vi "Initialize Control.vi"(8 "error in (no error)":errorcluster, 11 "DataGrid in":refnum<class "DataGrid.lvclass">) -> (0 "error out":errorcluster, 3 "DataGrid out":refnum<class "DataGrid.lvclass">)   [LabVIEW 2018, in "DataGrid.lvclass"]
doc: "The <b>Initialize VI</b> is a dynamic dispatch VI that must be overwritten in every QControl Class. It must <b>Call Parent Method</b> so that it recursively calls the initialize routine all of the way up the inheritance hierarchy. \n\nThe top most call is to the <b>Initialize Control VI</b> in Control.lvclass. This is the VI that starts the <b>Event Handler VI</b> if there was one overwritten in the QControl.\n<b> </b> <b> </b>\n©2016 Q Software Innovations, LLC (QSI)\nwritten by Quentin Alldredge\nproduced in LabVIEW 2015\n\nsupport@qsoftwareinnovations.com\nwww.qsoftwareinnovations.com\n\nAll rights reserved.\n\nRedistribution and use in source and binary forms, with or without modification, are permitted provided that the following conditions are met:\n\n * Redistributions of source code must retain the above copyright notice, this list of conditions and the following disclaimer.\n * Redistributions in binary form must reproduce the above copyright notice, this list of conditions and the following disclaimer in the documentation and/or other materials provided with the distribution.\n * Neither the name of Q Software Innovations, LLC. nor the names of its contributors may be used to endorse or promote products derived from this software without specific prior written permission.\n\nTHIS SOFTWARE IS PROVIDED BY THE COPYRIGHT HOLDERS AND CONTRIBUTORS \"AS IS\" AND ANY EXPRESS OR IMPLIED WARRANTIES, INCLUDING, BUT NOT LIMITED TO, THE IMPLIED WARRANTIES OF MERCHANTABILITY AND FITNESS FOR A PARTICULAR PURPOSE ARE DISCLAIMED. IN NO EVENT SHALL THE COPYRIGHT OWNER OR CONTRIBUTORS BE LIABLE FOR ANY DIRECT, INDIRECT, INCIDENTAL, SPECIAL, EXEMPLARY, OR CONSEQUENTIAL DAMAGES (INCLUDING, BUT NOT LIMITED TO, PROCUREMENT OF SUBSTITUTE GOODS OR SERVICES; LOSS OF USE, DATA, OR PROFITS; OR BUSINESS INTERRUPTION) HOWEVER CAUSED AND ON ANY THEORY OF LIABILITY, WHETHER IN CONTRACT, STRICT LIABILITY, OR TORT (INCLUDING NEGLIGENCE OR OTHERWISE) ARISING IN ANY WAY OUT OF THE USE OF THIS SOFTWARE, EVEN IF ADVISED OF THE POSSIBILITY OF SUCH DAMAGE."
uses:
  DataGrid.lvclass
  C:/Program Files (x86)/National Instruments/LabVIEW 2018/vi.lib/QSI/QControls/QControl Classes/MulticolumnListbox/MulticolumnListbox.lvclass
  DataGrid.lvclass/DataGrid.ctl
  Write Configuration.vi
  <vilib>/QSI/QControls/QControl Classes/MulticolumnListbox/MulticolumnListbox.lvclass
  <vilib>/QSI/DataGrid Configuration/DataGrid Config/DataGrid Config.lvclass
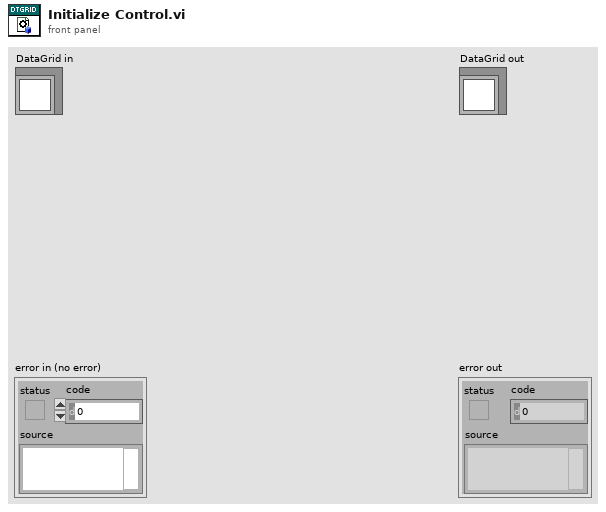
[diagram p1: front panel]
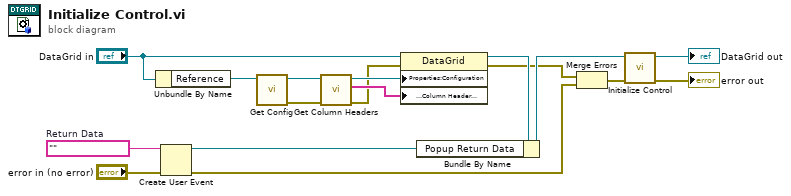
[diagram p0: block diagram]
diagram:
  w15 = ""  # Return Data
  n1 = Unbundle By Name("DataGrid in") -> ("Reference"=w10:refnum<vi>)
  n2 = Create User Event(user event datatype=w15, error in="error in (no error)") -> (user event=w14:refnum<user-event>, error out=w6:errorcluster)
  n3 = call <vilib>:"Get Config.vi"("Reference"=w10) -> ("error out"=w2:errorcluster, "DataGrid Config"=w5:refnum<class "DataGrid Config.lvclass">)  [unwired: 8 in, 1 out]
  n4 = call <vilib>:"Get Column Headers.vi"("error in (no error)"=w2, "DataGrid Config in"=w5) -> ("error out"=w1:errorcluster, "Column Headers[]"=w3:string[], "DataGrid Config out"=w4:refnum<class "DataGrid Config.lvclass">)  [unwired: 7 in]
  n5 = property class="DataGrid"(reference="DataGrid in", error in=w1, "Properties:Configuration"=w4, "Properties:Column Header Strings[]"=w3) -> (reference out=w9:refnum<class "DataGrid.lvclass">, error out=w8:errorcluster)
  n6 = Bundle By Name(cluster=w9, "Popup Return Data"=w14) -> (w13:refnum<class "DataGrid.lvclass">)
  n7 = Merge Errors(w8, w6) -> (w7:errorcluster)
  n8 = call-parent "Initialize Control.vi"("error in (no error)"=w7, "Control in"=w13) -> ("error out"=→"error out":errorcluster, "Control out"=→"DataGrid out":refnum<class "DataGrid.lvclass">)  [unwired: 8 in]
